vi "PCE_ANSWER-error-handler.vi"   [LabVIEW 2010]
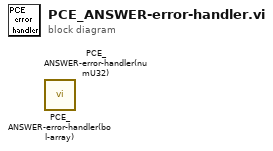
[diagram p0: block diagram]
diagram:
  n1 = call "PCE_ANSWER-error-handler(bol-array).vi"() -> ()  [unwired: 2 in, 1 out]
  n2 = call "PCE_ANSWER-error-handler(numU32).vi"() -> ()  [unwired: 2 in, 1 out]
